vi "IFD Sort Tags.vi"(8 "error in (no error)":errorcluster, 11 "IFD in":refnum<class "IFD.lvclass">) -> (0 "error out":errorcluster, 3 "IFD out":refnum<class "IFD.lvclass">)   [LabVIEW 2016, in "IFD.lvclass"]
uses:
  IFD.lvclass
  IFD.lvclass/IFD.ctl
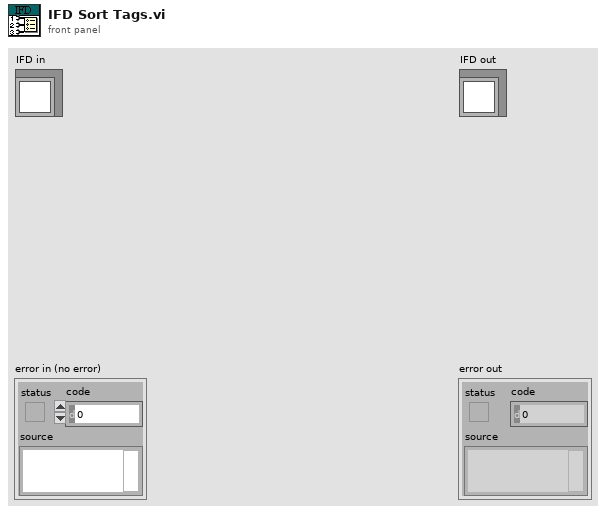
[diagram p1: front panel]
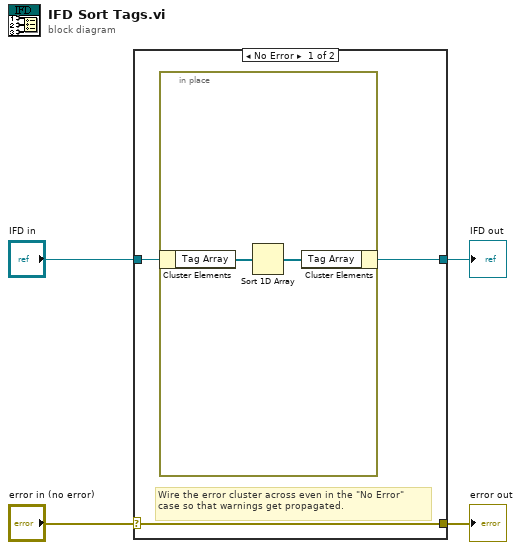
[diagram p0: block diagram]
diagram:
  n1 = case shown="No Error" "error in (no error)" {
    selector: "error in (no error)" -> [w7 w11]
    tunnel: [w7 w11] -> w3
    tunnel: [w5 w10] -> w1
    tunnel: "IFD in" -> [w6 w10]
    frame No Error {
      # "Wire the error cluster across even in the \"No Error\"\ncase so that warnings get propagated."
      n2 = in-place {
        n3 = in-place-cluster #1(w6) -> ("Tag Array"=w9:refnum<class "IFD_Tag.lvclass">[])
        n4 = Sort 1D Array(array=w9) -> (sorted array=w8:refnum<class "IFD_Tag.lvclass">[])
        n5 = in-place-cluster #1("Tag Array"=w8) -> (w5:refnum<class "IFD.lvclass">)
      }
    }
    frame Error {
    }
  }
  "error out" <- w3
  "IFD out" <- w1
